vi "Missing System Graphs 1.vi"() -> ()   [LabVIEW 2009]
panel:
  out "System Waveform Graph":dbl[](graph)
  out "System XY Graph":cluster{dbl, dbl}[](graph)
  out "System Waveform Chart":dbl(graph)
  out "System Intensity Chart":dbl[][](graph)
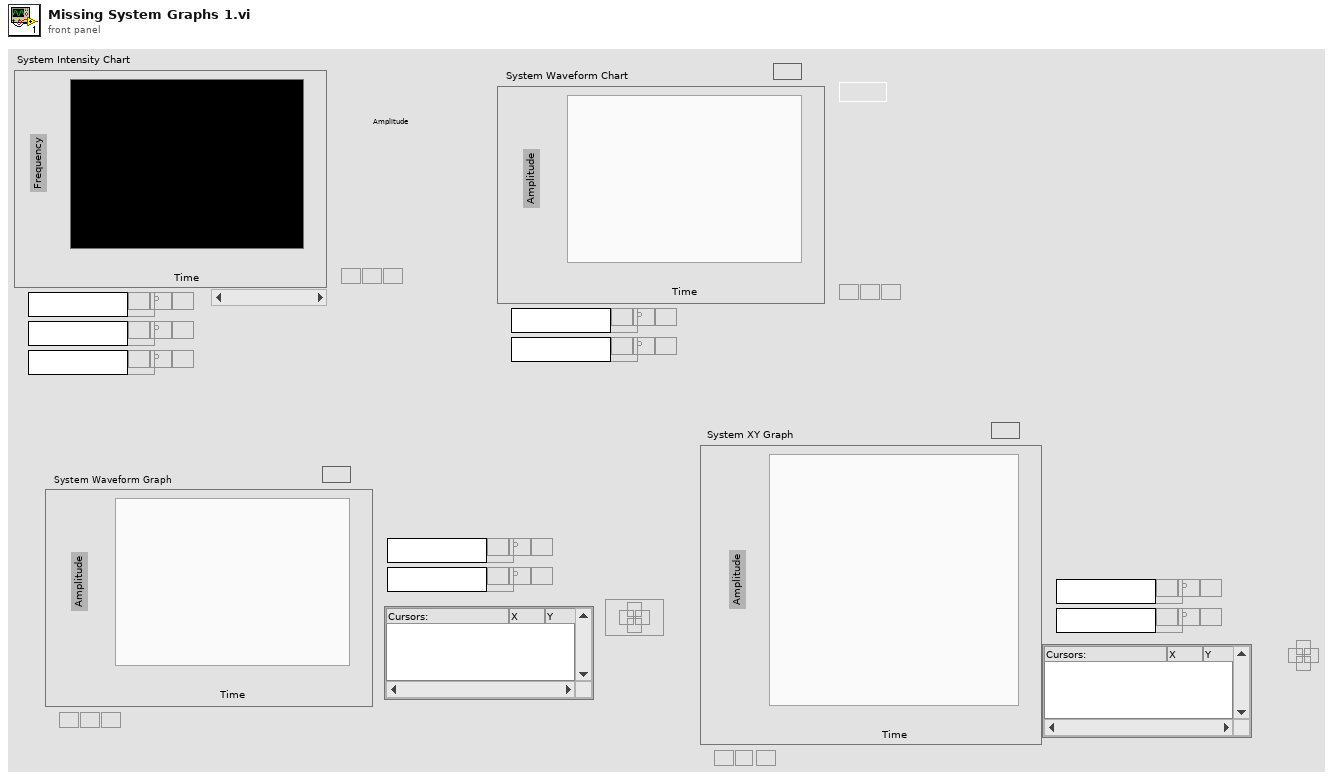
[diagram p1: front panel]
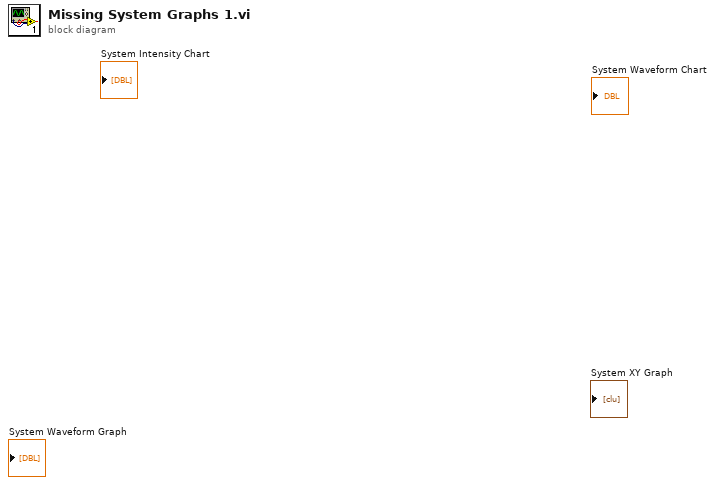
[diagram p0: block diagram]
diagram:
